vi "Construct Serializable Account.vi"(5 "Serializable Account in":refnum<class "Serializable Account.lvclass">, 7 "Roles":string[](array[string]), 8 "error in (no error)":errorcluster, 9 "CreatedDate":timestamp, 10 "Active":bool, 11 "Email":string) -> (0 "error out":errorcluster, 3 "Serializable Account":refnum<class "Serializable Account.lvclass">)   [LabVIEW 2017, in "Serializable Account.lvclass"]
uses:
  Serializable Account.lvclass
  Serializable Account.lvclass/Serializable Account.ctl
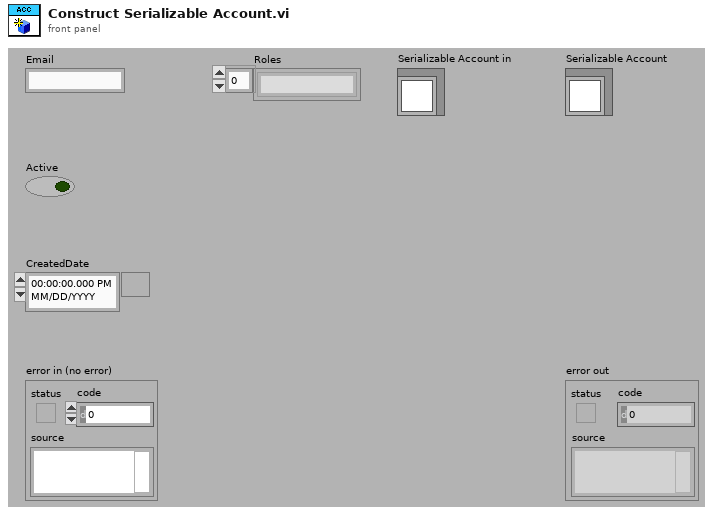
[diagram p1: front panel]
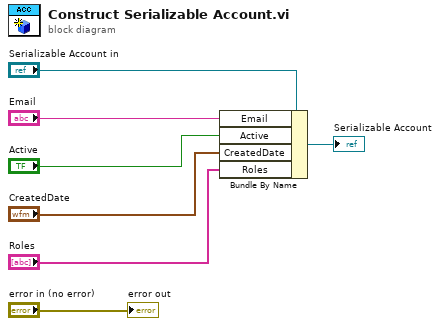
[diagram p0: block diagram]
diagram:
  n1 = Bundle By Name(cluster="Serializable Account in", "Email"="Email", "Active"="Active", "CreatedDate"="CreatedDate", "Roles"="Roles") -> (→"Serializable Account":refnum<class "Serializable Account.lvclass">)
  "error out" <- "error in (no error)"
